vi "Set to VArray.vi"(8 "error in":errorcluster, 11 "Set":variant) -> (0 "error out":errorcluster, 3 "Array":variant)   [LabVIEW 2020, in "openg_variant.lvlib"]
uses:
  openg_variant.lvlib
panel:
  # "EXPERIMENTAL"
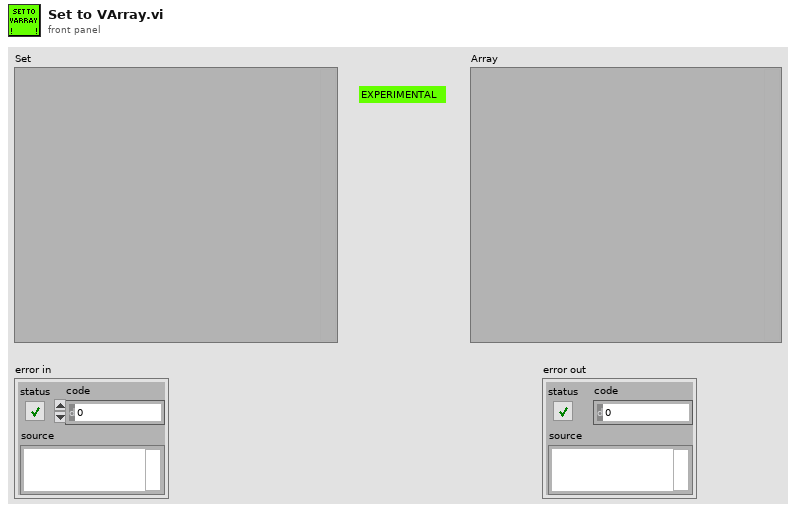
[diagram p1: front panel]
types:
  T1 = typedef "openg_variant.lvlib/Type Descriptor.ctl" = i16[]
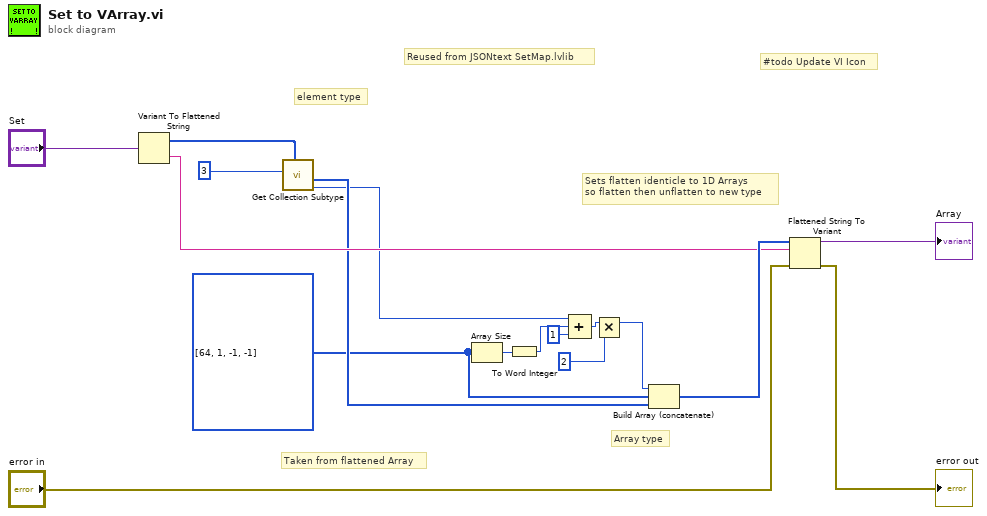
[diagram p0: block diagram]
diagram:
  w12 = i16[] [64, 1, -1, -1] ("type string 7")
  # "#todo Update VI Icon"
  # "Taken from flattened Array"
  # "Sets flatten identicle to 1D Arrays\nso flatten then unflatten to new type"
  # "element type"
  # "Array type"
  # "Reused from JSONtext SetMap.lvlib"
  n1 = Variant To Flattened String(Variant="Set") -> (data string=w14:string, 1:w5:i16[])
  n2 = call "Get Collection Subtype.vi"("Type Descriptor"=w5, "Offset In"=i16 3 ("index")) -> ("Size"=w6:i16, "subtype"=w13:T1)  [unwired: 7 in, 1 out]
  n3 = Array Size(array=w12) -> (size(s)=w11:i32)
  n4 = To Word Integer(number=w11) -> (16bit integer=w9:i16)
  n5 = Compound Arithmetic op=ADD(w6, w9, i16 1 ("value")) -> (w10:i16)
  n6 = Multiply(x=w10, y=i16 2) -> (x*y=w16:i16)
  n7 = Build Array (concatenate)(w16, w12, w13) -> (w15:T1)
  n8 = Flattened String To Variant(4:"error in", 6:w14, 7:w15) -> (0:→"error out":errorcluster, 3:→"Array":variant)
